vi "wd_addRecordInOneNode (Time).vi"(6 "length":u64, 7 "data":timestamp[](array[timestamp]), 8 "error in (no error)":errorcluster, 9 "start":u64, 10 "datalog postion":i64, 11 "meta in":T1={"TargetFile"=path "", "StreamMode"=enum."File", "Append?"=FALSE, "ChunkSize"=0, "TimeColumnMode"=enum."Empty", "TimestampFormat"="", "AbsoluteTime?"=FALSE, "FileAttribute "={"Creator"="", "Title"="", "SheetName"=""}, "Column"=[], "FileRef"=refnum, "MemoryRef"=[], "RecordInfo"=[], " ChannelPreviousInfo"=[], "ChannelFirstRecord"=[], "PredefinedFormattedValueLength"=20, "DiskTemplate"={"XMLRef"=[refnum, refnum, refnum, refnum, refnum, refnum], "ZipPath"=path "", "MetaFile"={"Ref"=refnum, "NextRow"=0, "NextPosition"=0, "Block"=[]}, "TempFolder"=path ""}}) -> (0 "error out":errorcluster, 3 "meta out":T1={"TargetFile"=path "", "StreamMode"=enum."File", "Append?"=FALSE, "ChunkSize"=0, "TimeColumnMode"=enum."Empty", "TimestampFormat"="", "AbsoluteTime?"=FALSE, "FileAttribute "={"Creator"="", "Title"="", "SheetName"=""}, "Column"=[], "FileRef"=refnum, "MemoryRef"=[], "RecordInfo"=[], " ChannelPreviousInfo"=[], "ChannelFirstRecord"=[], "PredefinedFormattedValueLength"=20, "DiskTemplate"={"XMLRef"=[refnum, refnum, refnum, refnum, refnum, refnum], "ZipPath"=path "", "MetaFile"={"Ref"=refnum, "NextRow"=0, "NextPosition"=0, "Block"=[]}, "TempFolder"=path ""}}, 4 "data subset":timestamp[](array[timestamp]))   [LabVIEW 2020, in "NI_ExcelFile.lvlib"]
uses:
  <vilib>/express/express shared/NI_ExcelFile/NI_ExcelFile.lvlib
  <vilib>/express/express shared/NI_ExcelFile/Ctrls/MainData.ctl
  <vilib>/express/express shared/NI_ExcelFile/Ctrls/StreamMode.ctl
  <vilib>/express/express shared/NI_ExcelFile/Ctrls/TimeColumnMode.ctl
  <vilib>/express/express shared/NI_ExcelFile/Ctrls/FileAttribute.ctl
  <vilib>/express/express shared/NI_ExcelFile/Ctrls/Columns.ctl
  <vilib>/express/express shared/NI_ExcelFile/Ctrls/ColumnInfo.ctl
  <vilib>/express/express shared/NI_ExcelFile/Ctrls/DataType.ctl
  <vilib>/express/express shared/NI_ExcelFile/Ctrls/wd_recordInfo.ctl
  <vilib>/express/express shared/NI_ExcelFile/Ctrls/disk_TemplateFile.ctl
  <vilib>/express/express shared/NI_ExcelFile/Ctrls/meta_file.ctl
  <vilib>/express/express shared/NI_ExcelFile/Ctrls/meta_Block.ctl
  <vilib>/express/express shared/NI_ExcelFile/Ctrls/meta_BlockType.ctl
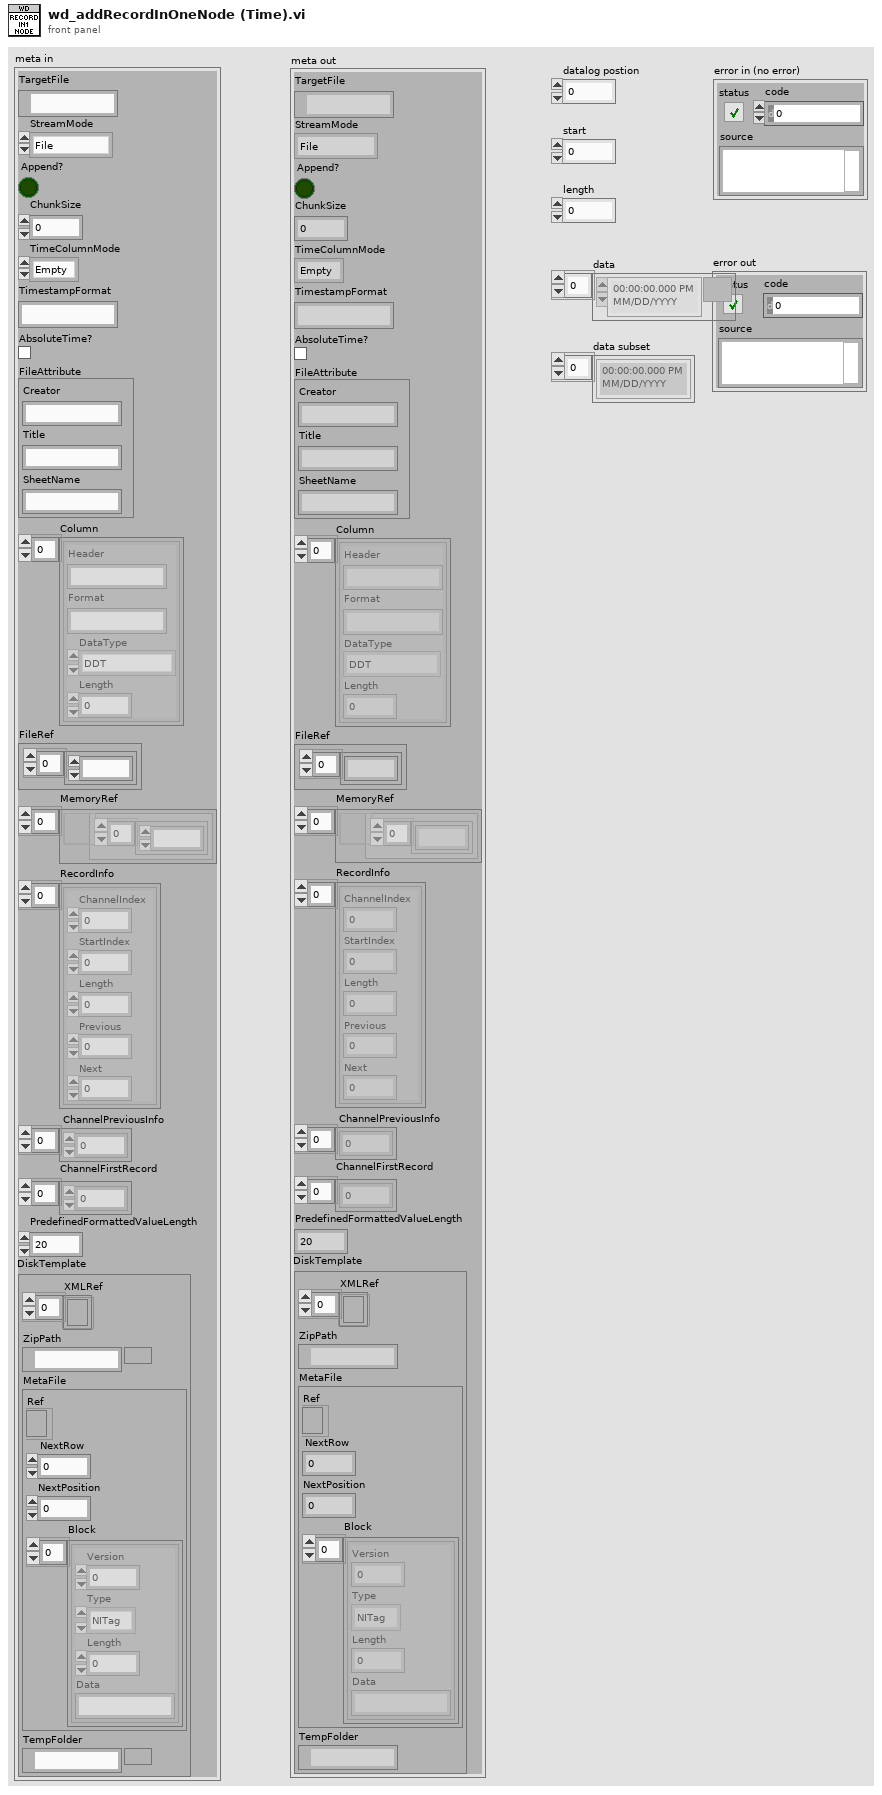
[diagram p1: front panel]
types:
  T1 = typedef "NI_ExcelFile.lvlib/MainData.ctl" = cluster{"TargetFile":path, "StreamMode":T2, "Append?":bool, "ChunkSize":u64, "TimeColumnMode":T3, "TimestampFormat":string, "AbsoluteTime?":bool, "FileAttribute ":T4, "Column":T5, "FileRef":refnum<k1>, "MemoryRef":refnum<data-value>[], "RecordInfo":T8[], " ChannelPreviousInfo":u32[], "ChannelFirstRecord":u32[], "PredefinedFormattedValueLength":i64, "DiskTemplate":T9}
  T2 = typedef "NI_ExcelFile.lvlib/StreamMode.ctl" = enum16{"File", "Memory"}
  T3 = typedef "NI_ExcelFile.lvlib/TimeColumnMode.ctl" = enum16{"Empty", "OnePerCh", "One"}
  T4 = typedef "NI_ExcelFile.lvlib/FileAttribute.ctl" = cluster{"Creator":string, "Title":string, "SheetName":string}
  T5 = typedef "NI_ExcelFile.lvlib/Columns.ctl" = T6[]
  T6 = typedef "NI_ExcelFile.lvlib/ColumnInfo.ctl" = cluster{"Header":string, "Format":string, "DataType":T7, "Length":u64}
  T7 = typedef "NI_ExcelFile.lvlib/DataType.ctl" = enum16{"DDT", "WFM", "Array of STR", "Array of DBL", "Array of I8", "Array of I16", "Array of I32", "Array of I64", "Array of SGL", "Array of U8", "Array of U16", "Array of U32", "Array of U64", "Array of Time"}
  T8 = typedef "NI_ExcelFile.lvlib/wd_recordInfo.ctl" = cluster{"ChannelIndex":u32, "StartIndex":u64, "Length":u64, "Previous":i32, "Next":i32}
  T9 = typedef "NI_ExcelFile.lvlib/disk_TemplateFile.ctl" = cluster{"XMLRef":refnum<file>[], "ZipPath":path, "MetaFile":T10, "TempFolder":path}
  T10 = typedef "NI_ExcelFile.lvlib/meta_file.ctl" = cluster{"Ref":refnum<file>, "NextRow":i32, "NextPosition":i64, "Block":T11[]}
  T11 = typedef "NI_ExcelFile.lvlib/meta_Block.ctl" = cluster{"Version":u16, "Type":T12, "Length":i32, "Data":string}
  T12 = typedef "NI_ExcelFile.lvlib/meta_BlockType.ctl" = enum16{"NITag", "File", "Column"}
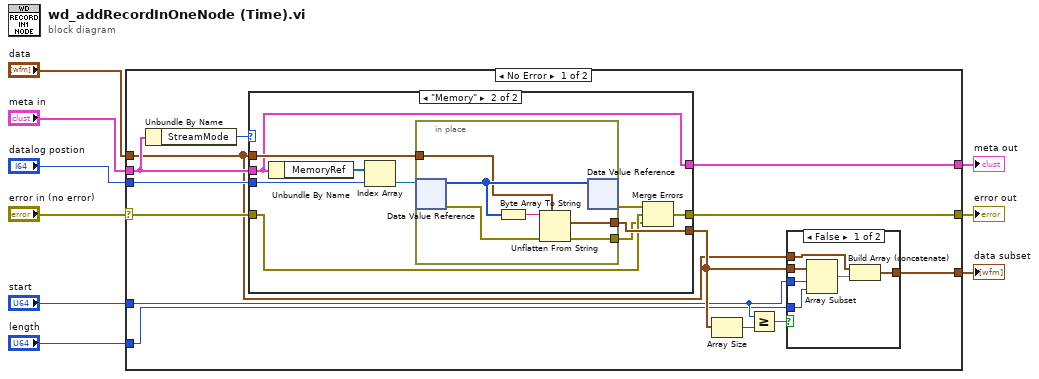
[diagram p0: block diagram]
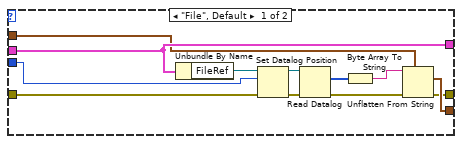
[diagram p3: hidden frame]
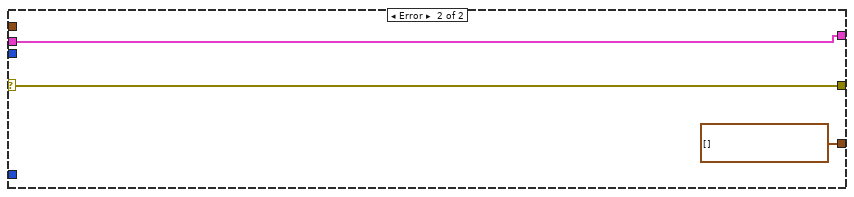
[diagram p4: hidden frame]
diagram:
  n1 = case shown="No Error" "error in (no error)" {
    selector: "error in (no error)" -> [w18 w59]
    tunnel: "datalog postion" -> [w17 _]
    tunnel: [w10 timestamp[] [] ("data")] -> w8
    tunnel: "meta in" -> [w19 w60]
    tunnel: [w13 w60] -> w6
    tunnel: [w12 w59] -> w5
    tunnel: "data" -> [w11 _]
    tunnel: "start" -> [w15 _]
    tunnel: "length" -> [w14 _]
    frame No Error {
      n2 = Unbundle By Name(w19) -> ("StreamMode"=w22:T2)
      n3 = case shown="\"Memory\"" w22 {
        tunnel: w19 -> [w33 w47]
        tunnel: w18 -> [w35 w44]
        tunnel: w17 -> [w37 w48]
        tunnel: [w33 w47] -> w13
        tunnel: w11 -> [w32 w50]
        tunnel: [w31 w46] -> w16
        tunnel: [w30 w42] -> w12
        frame "File", Default {
          n4 = Unbundle By Name(w33) -> ("FileRef"=w36:refnum<k1>)
          n5 = Set Datalog Position(4:w35, 6:w37, 7:w36) -> (0:w41:errorcluster, 3:w38:refnum<k1>)  [unwired: 1 in]
          n6 = Read Datalog(4:w41, 7:w38) -> (0:w34:errorcluster, 2:w39:u8[])  [unwired: 1 in, 1 out]
          n7 = Byte Array To String(unsigned byte array=w39) -> (string=w40:string)
          n8 = Unflatten From String(type=w32, binary string=w40, error in (no error)=w34) -> (value=w31:timestamp[], error out=w30:errorcluster)  [unwired: 2 in, 1 out]
        }
        frame "Memory" {
          n9 = Unbundle By Name(w47) -> ("MemoryRef"=w49:refnum<data-value>[])
          n10 = Index Array(array=w49, index=w48) -> (element=w51:refnum<data-value>)
          n11 = in-place {
            in-place-border: w50 -> [w54]
            in-place-border: [w53] -> w46
            in-place-border: [w52] -> w43
            n12 = in-place-dvr #1(w51) -> (w56:u8[], w55:errorcluster)
            n13 = Byte Array To String(unsigned byte array=w56) -> (string=w57:string)
            n14 = Unflatten From String(type=w54, binary string=w57, error in (no error)=w55) -> (value=w53:timestamp[], error out=w52:errorcluster)  [unwired: 2 in, 1 out]
            n15 = in-place-dvr #1(w56) -> (w45:errorcluster)  [unwired: 1 out]
          }
          n16 = Merge Errors(w45, w44, w43) -> (w42:errorcluster)
        }
      }
      n17 = Array Size(array=w16) -> (size(s)=w21:i32)
      n18 = Greater Or Equal?(x=w15, y=w21) -> (x >= y?=w20:bool)
      n19 = case shown="False" w20 {
        tunnel: w16 -> [w28 _]
        tunnel: w15 -> [w27 _]
        tunnel: w14 -> [w26 _]
        tunnel: w11 -> [w25 w29]
        tunnel: [w23 w29] -> w10
        frame False {
          n20 = Array Subset(array=w28, index=w27, length=w26) -> (w24:timestamp[])
          n21 = Build Array (concatenate)(w25, w24) -> (w23:timestamp[])
        }
        frame True {
        }
      }
    }
    frame Error {
    }
  }
  "data subset" <- w8
  "meta out" <- w6
  "error out" <- w5
